vi "Backup File.vi"(8 "Error In":errorcluster, 9 "Suffix?":bool, 10 "Prefix":string="BAC_", 11 "File":path) -> (0 "Error Out":errorcluster, 2 "Back-up file":path, 3 "Duplicate file":path)   [LabVIEW 2018]
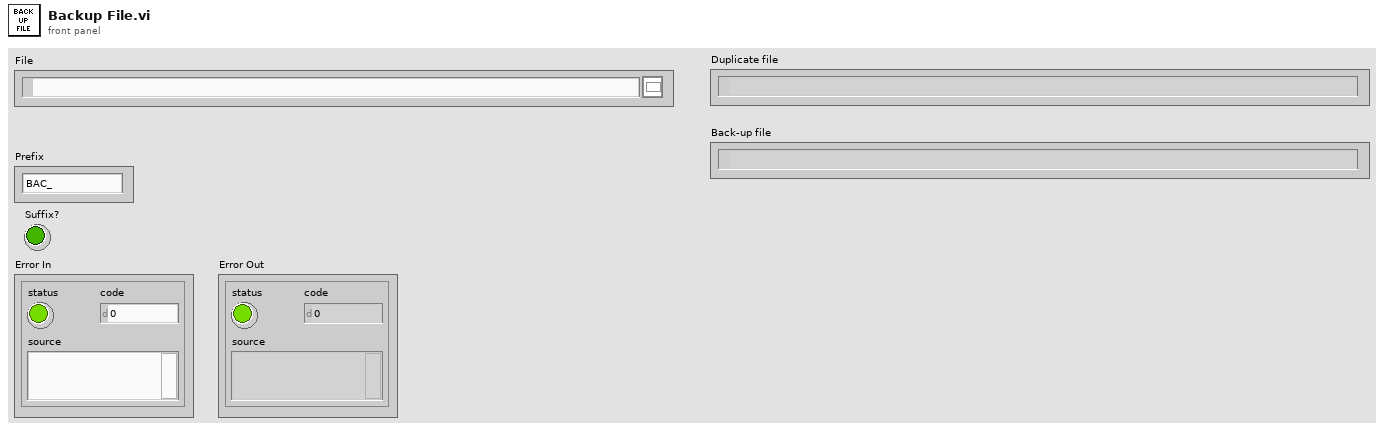
[diagram p1: front panel]
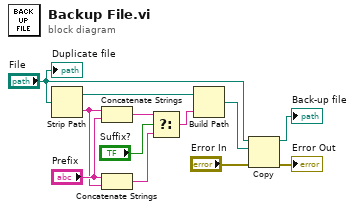
[diagram p0: block diagram]
diagram:
  n1 = Strip Path(path="File") -> (stripped path=w11:path, name=w3:string)
  n2 = Concatenate Strings(w3, "Prefix") -> (w5:string)
  n3 = Concatenate Strings("Prefix", w3) -> (w2:string)
  n4 = Select(t=w5, s="Suffix?", f=w2) -> (s? t:f=w1:string)
  n5 = Build Path(base path=w11, name or relative path=w1) -> (appended path=w10:path)
  n6 = Copy(8:"Error In", 10:w10, 11:"File") -> (0:→"Error Out":errorcluster, 3:→"Back-up file":path)  [unwired: 2 in, 1 out]
  "Duplicate file" <- "File"
